vi "Get Array False Details.vi"(11 "Array":bool[](array[boolean])) -> (2 "First False":i32, 3 "Count":i16)   [LabVIEW 2015, in "VITAC.lvlib"]
uses:
  VITAC.lvlib
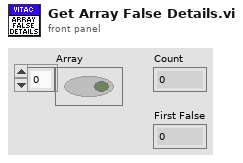
[diagram p1: front panel]
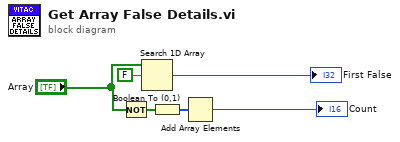
[diagram p0: block diagram]
diagram:
  n1 = Not(x="Array") -> (.not. x?=w5:bool[])
  n2 = Search 1D Array(1D array="Array", element=FALSE) -> (index of element=→"First False":i32)  [unwired: 1 in]
  n3 = Boolean To (0,1)(Boolean=w5) -> (0, 1=w2:i16[])
  n4 = Add Array Elements(numeric array=w2) -> (sum=→"Count":i16)
